vi "Read(Y)Trace.vi"(8 "error in (no error)":errorcluster, 11 "Keysight44xx in":refnum<class "Keysight44xx.lvclass">) -> (0 "error out":errorcluster, 2 "Waveform(s)":T1, 3 "Keysight44xx out":refnum<class "Keysight44xx.lvclass">)   [LabVIEW 2018, in "SpecAnPlugins.lvlib" / "Keysight44xx.lvclass"]
doc: "This function initiates a signal acquisition based on the present instrument configuration. It then waits for the acquisition to complete, and returns the trace as an array of amplitude values. The amplitude array returns data that represent the amplitude of the signals obtained by sweeping from the start frequency to the stop frequency (in frequency domain, in time domain the amplitude array is ordered from beginning of sweep to end). The Amplitude Units attribute determines the units of the points in the amplitude array. This function resets the sweep count.\n\nIf the spectrum analyzer did not complete the acquisition within the time period the user specified with the MaxTime parameter, the function returns the Max Time Exceeded error."
uses:
  Keysight44xx.lvclass
  C:/Users/ico/Documents/Projects/NistPluggableModules/SpecAn/SpecAnPlugins/SpecAnBaseClass/SpecAnBase.lvclass
  SpecAnBaseClass/Typedefs/Waveform(s).ctl
  SpecAnBaseClass/SpecAnBase.lvclass
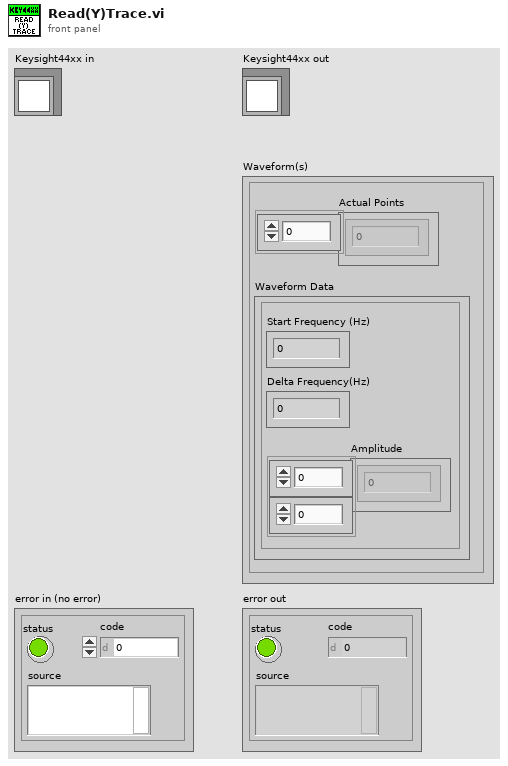
[diagram p1: front panel]
types:
  T1 = typedef "SpecAnPlugins.lvlib/SpecAnBase.lvclass/Waveform(s).ctl" = cluster{"Actual Points":i32[], "Waveform Data":cluster{"Start Frequency (Hz)":dbl, "Delta Frequency(Hz)":dbl, "Amplitude":dbl[][]}}
  T2 = typedef "SpecAnPlugins.lvlib/SpecAnBase.lvclass/Acquisition.ctl" = cluster{"Handle":string, "Connected":bool, "Enabled":bool, "SweepModeContinuous":bool, "NumberOfSweeps":i32, "DetectorTypeAuto":bool, "DetectorType":i32, "VerticalScale":i32, "MaximumTime(seconds)":dbl}
  T3 = typedef "SpecAnPlugins.lvlib/SpecAnBase.lvclass/Trace.ctl" = cluster{"TraceName":string, "TraceSize":i32, "TraceType":i32}[]
  T4 = typedef "SpecAnPlugins.lvlib/SpecAnBase.lvclass/Frequency.ctl" = cluster{"FrequencyStart":dbl, "FrequencyStop":dbl, "FrequencyOffset":dbl}
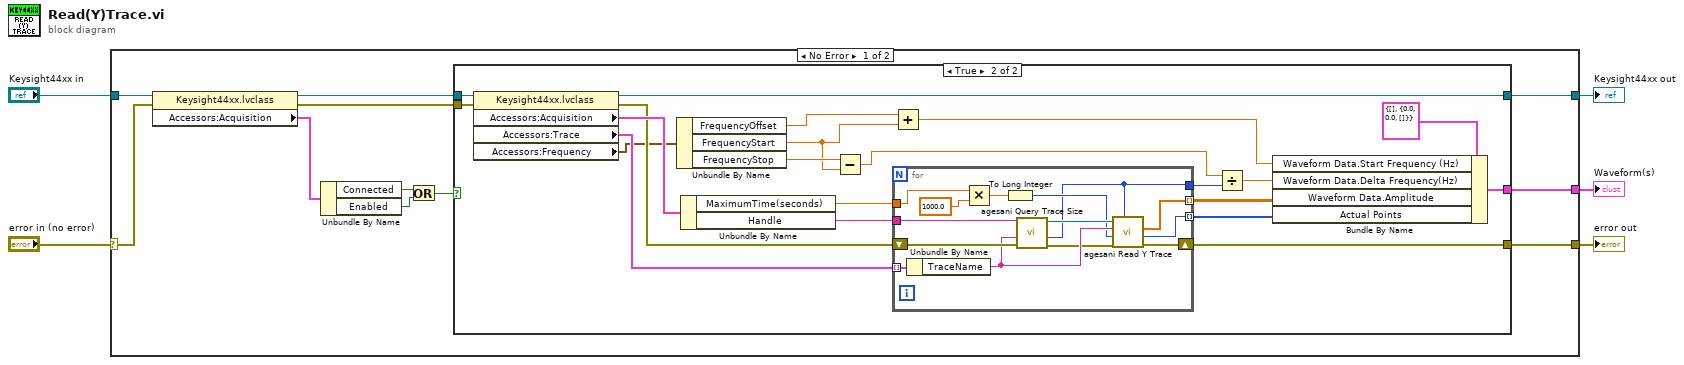
[diagram p0: block diagram]
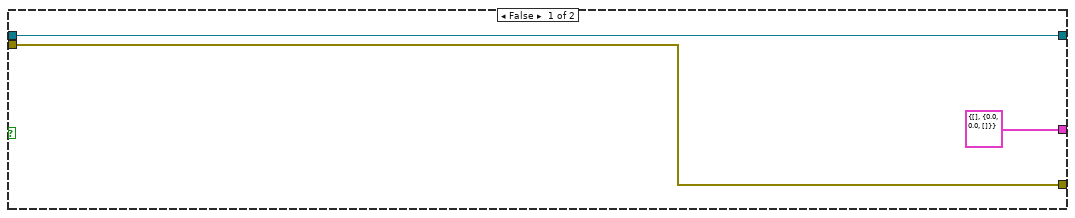
[diagram p2: hidden frame]
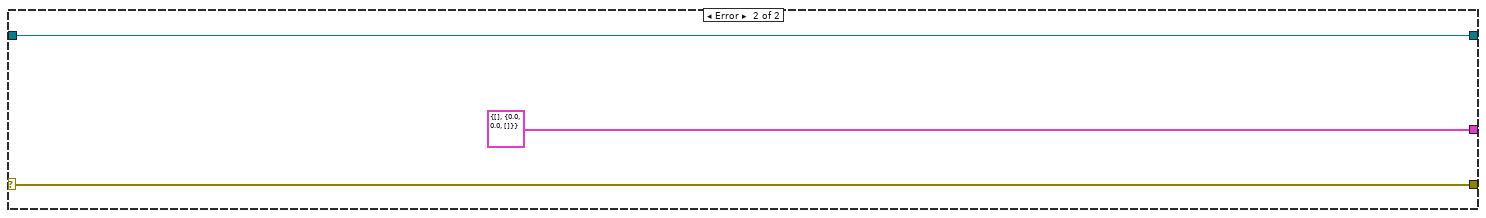
[diagram p3: hidden frame]
diagram:
  n1 = case shown="No Error" "error in (no error)" {
    selector: "error in (no error)" -> [w11 w57]
    tunnel: [w15 w57] -> w4
    tunnel: "Keysight44xx in" -> [w12 w56]
    tunnel: [w16 w56] -> w2
    tunnel: [w14 T1 {"Actual Points"=[], "Waveform Data"={"Start Frequency (Hz)"=0.0, "Delta Frequency(Hz)"=0.0, "Amplitude"=[]}} ("Waveform(s)")] -> w1
    frame No Error {
      n2 = property class="Keysight44xx.lvclass"(reference=w12, error in=w11) -> (reference out=w9:refnum<class "Keysight44xx.lvclass">, error out=w10:errorcluster, "Accessors:Acquisition"=w13:T2)
      n3 = Unbundle By Name(w13) -> ("Connected"=w8:bool, "Enabled"=w7:bool)
      n4 = Or(x=w8, y=w7) -> (x .or. y?=w6:bool)
      n5 = case shown="True" w6 {
        tunnel: [w19 w40] -> w16
        tunnel: [w18 w37] -> w15
        tunnel: [T1 {"Actual Points"=[], "Waveform Data"={"Start Frequency (Hz)"=0.0, "Delta Frequency(Hz)"=0.0, "Amplitude"=[]}} ("Waveform(s)") w32] -> w14
        tunnel: w10 -> [w18 w21]
        tunnel: w9 -> [w19 w20]
        frame False {
        }
        frame True {
          n6 = property class="Keysight44xx.lvclass"(reference=w20, error in=w21) -> (reference out=w40:refnum<class "Keysight44xx.lvclass">, error out=w36:errorcluster, "Accessors:Acquisition"=w39:T2, "Accessors:Trace"=w35:T3, "Accessors:Frequency"=w29:T4)
          n7 = Unbundle By Name(w29) -> ("FrequencyOffset"=w24:dbl, "FrequencyStart"=w23:dbl, "FrequencyStop"=w28:dbl)
          n8 = Unbundle By Name(w39) -> ("MaximumTime(seconds)"=w34:dbl, "Handle"=w38:string)
          n9 = Subtract(x=w28, y=w23) -> (x-y=w26:dbl)
          n10 = Add(x=w24, y=w23) -> (x+y=w22:dbl)
          n11 = for {
            tunnel: w38 -> [w52]
            shift-right: [w54] -> w37
            shift-left: w36 -> [w51]
            tunnel: w35 -> [w53] mode=indexing
            tunnel: w34 -> [w45]
            tunnel: [w47] -> w30 mode=indexing
            tunnel: [w46] -> w31 mode=indexing
            tunnel: [w41] -> w27
            n12 = Unbundle By Name(w53) -> ("TraceName"=w50:string)
            n13 = Multiply(x=w45, y=1000.0) -> (x*y=w43:dbl)
            n14 = To Long Integer(number=w43) -> (32bit integer=w42:i32)
            n15 = call <instrlib>:"agesani Query Trace Size.vi"("error in (no error)"=w51, "trace name (\"\")"=w50, "instrument handle"=w52) -> ("error out"=w49:errorcluster, "trace size"=w41:i32, "instrument handle out"=w48:refnum<k15>)  [unwired: 6 out]
            n16 = call <instrlib>:"agesani Read Y Trace.vi"("array length"=w41, "error in (no error)"=w49, "maximum time"=w42, "trace name"=w50, "instrument handle"=w48) -> ("error out"=w54:errorcluster, "actual points"=w46:i32, "amplitude"=w47:dbl[])  [unwired: 3 in, 1 out]
          }
          n17 = Divide(x=w26, y=w27) -> (x/y=w25:dbl)
          n18 = Bundle By Name(cluster=T1 {"Actual Points"=[], "Waveform Data"={"Start Frequency (Hz)"=0.0, "Delta Frequency(Hz)"=0.0, "Amplitude"=[]}} ("Waveform(s)"), "Waveform Data.Start Frequency (Hz)"=w22, "Waveform Data.Delta Frequency(Hz)"=w25, "Waveform Data.Amplitude"=w30, "Actual Points"=w31) -> (w32:T1)
        }
      }
    }
    frame Error {
    }
  }
  "error out" <- w4
  "Keysight44xx out" <- w2
  "Waveform(s)" <- w1
